vi "数据全参数一起发送整点触发.vi"(6 "数据发送通道":enum16{"TCP", "VISA"}(ring), 8 "PW":string, 9 "MN":string) -> ()   [LabVIEW 2016, in "数据传输系统.lvlib"]
panel:
  out "table":string="提取小时数据"
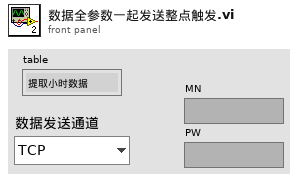
[diagram p1: front panel]
types:
  T1 = typedef "LVDateTimeRec.ctl" = cluster{"秒数的小数部分":dbl, "秒":i32, "分":i32, "时":i32, "日":i32, "月":i32, "年":i32, "天数（周）":i32, "天数（年）":i32, "DST":i32}
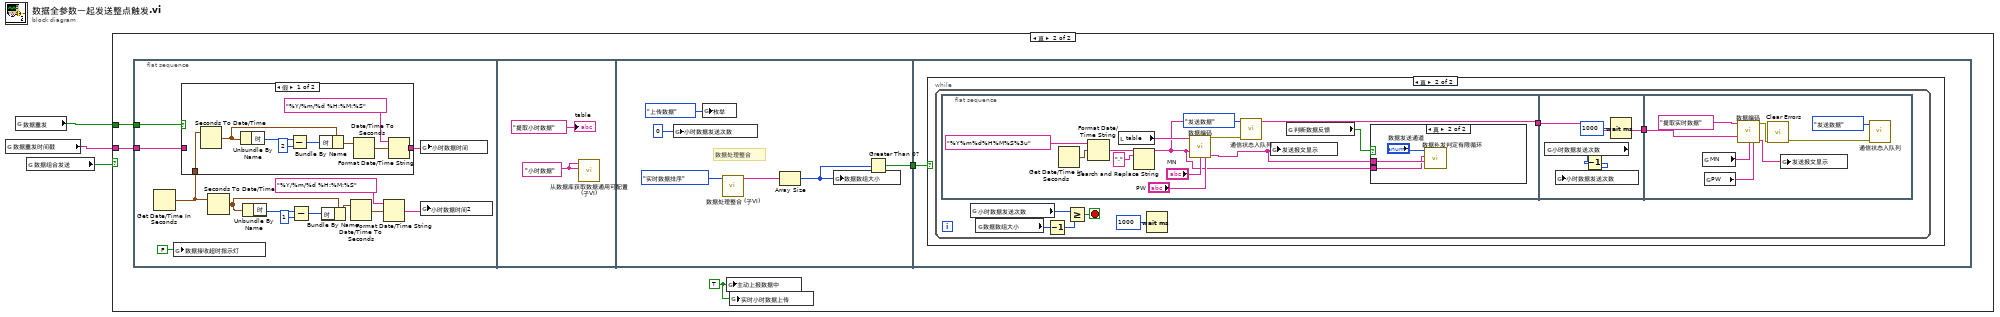
[diagram p0: block diagram]
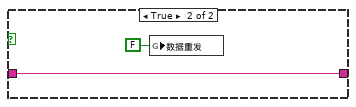
[diagram p3: hidden frame]
diagram:
  n1 = global read "断电保存全局.vi" "数据重发时间戳"() -> (w1:string)
  n2 = global read "断电保存全局.vi" "数据重发"() -> (w2:bool)
  n3 = global read "断电保存全局.vi" "数据组合发送"() -> (w3:bool)
  n4 = case shown="真" w3 {
    tunnel: w2 -> [_ w6]
    tunnel: w1 -> [_ w5]
    frame False {
    }
    frame True {
      w4 = TRUE ("主动上报数据中")
      n5 = flat-sequence {
        tunnel: w6 -> [w15]
        tunnel: w5 -> [w14]
        tunnel: [w35] -> w7
        tunnel: w7 -> [w40]
        frame #0 {
          n6 = Get Date/Time In Seconds() -> (seconds since 1Jan1904=w20:timestamp)
          n7 = global write "全局 数据发送重叠.vi" "数据接收超时指示灯"(FALSE ("数据接收超时指示灯")) -> ()
          n8 = case shown="假" w15 {
            tunnel: w20 -> [w29 _]
            tunnel: [w21 w31] -> w17
            tunnel: w14 -> [_ w31]
            frame False {
              n9 = Seconds To Date/Time(time stamp (now)=w29) -> (date time rec=w24:T1)  [unwired: 1 in]
              n10 = Unbundle By Name(w24) -> ("时"=w22:i32)
              n11 = Subtract(x=w22, y=2) -> (x-y=w25:i32)
              n12 = Bundle By Name(cluster=w24, "时"=w25) -> (w26:T1)
              n13 = Date/Time To Seconds(2:w26) -> (0:w27:timestamp)  [unwired: 1 in]
              n14 = Format Date/Time String(time format string (%c)="%Y/%m/%d %H:%M:%S" ("时间格式字符串(%c)"), seconds (now)=w27) -> (date/time string=w21:string)  [unwired: 1 in]
            }
            frame True {
              n15 = global write "断电保存全局.vi" "数据重发"(FALSE ("数据重发")) -> ()
            }
          }
          n16 = Seconds To Date/Time(time stamp (now)=w20) -> (date time rec=w10:T1)  [unwired: 1 in]
          n17 = Unbundle By Name(w10) -> ("时"=w13:i32)
          n18 = Subtract(x=w13, y=1) -> (x-y=w11:i32)
          n19 = Bundle By Name(cluster=w10, "时"=w11) -> (w9:T1)
          n20 = Date/Time To Seconds(2:w9) -> (0:w19:timestamp)  [unwired: 1 in]
          n21 = Format Date/Time String(time format string (%c)="%Y/%m/%d %H:%M:%S" ("时间格式字符串(%c)"), seconds (now)=w19) -> (date/time string=w16:string)  [unwired: 1 in]
          n22 = global write "全局 时间2.vi" "小时数据时间2"(w16) -> ()
          n23 = global write "全局 水样时间.vi" "小时数据时间"(w17) -> ()
        }
        frame #1 {
          w33 = "小时数据" ("名称（未命名）")
          n24 = call "从数据库获取数据通用可配置(子VI).vi"("table输入"=w33, "列队名（唯一）"=w33) -> ()  [unwired: 8 in, 2 out]
          "table" <- "提取小时数据" ("新元素/子数组")
        }
        frame #2 {
          # "数据处理整合"
          n25 = global write "全局 小时数据发送次数.vi" "小时数据发送次数"(0 ("数值")) -> ()
          n26 = global write "全局1.vi" "枚举"(enum16{"返回请求应答", "上传数据", "返回执行结果"}."上传数据" ("枚举")) -> ()
          n27 = call "数据处理整合 (子VI).vi"("枚举"=enum16{"实时数据排序", "小时数据排序"}."实时数据排序") -> ("已排序的数组"=w39:string[])  [unwired: 10 in]
          n28 = Array Size(array=w39) -> (size(s)=w36:i32)
          n29 = global write "全局 数据数组大小.vi" "数据数组大小"(w36) -> ()
          n30 = Greater Than 0?(x=w36) -> (x > 0?=w35:bool)
        }
        frame #3 {
          n31 = case shown="真" w40 {
            frame False {
            }
            frame True {
              n32 = while {
                stop <- w46 stop-if-true
                n33 = flat-sequence {
                  tunnel: [w48] -> w42
                  tunnel: w42 -> [w66]
                  tunnel: [w66] -> w41
                  tunnel: w41 -> [w67]
                  frame #0 {
                    n34 = Get Date/Time In Seconds() -> (seconds since 1Jan1904=w54:timestamp)
                    n35 = Format Date/Time String(time format string (%c)="%Y%m%d%H%M%S%3u" ("时间格式字符串(%c)"), seconds (now)=w54) -> (date/time string=w55:string)  [unwired: 1 in]
                    n36 = local read "table"() -> (w59:string)
                    n37 = Search and Replace String(input string=w55, search string="." ("搜索字符串")) -> (result string=w48:string)  [unwired: 6 in, 3 out]
                    n38 = call "数据编码.vi"("table输入"=w59, "QN"=w48, "MN"="MN", "PW"="PW") -> ("错误常量"=w49:errorcluster, "通讯包字符串"=w51:string)  [unwired: 10 in]
                    n39 = call "通信状态入队列.vi"("错误输入（无错误）"=w49, "枚举"=enum16{"打开连接", "发送数据", "读取数据", "数据处理", "关闭连接"}."发送数据") -> ()  [unwired: 9 in, 1 out]
                    n40 = global write "全局1.vi" "发送报文显示"(w51) -> ()
                    n41 = global read "断电保存全局.vi" "判断数据反馈"() -> (w52:bool)
                    n42 = case shown="真" w52 {
                      tunnel: w51 -> [_ w62]
                      tunnel: w48 -> [_ w60]
                      frame False {
                      }
                      frame True {
                        n43 = call "数据补发判定有限循环.vi"("数据输入"=w62, "QN"=w60, "数据发送通道"="数据发送通道") -> ()  [unwired: 8 in, 1 out]
                      }
                    }
                  }
                  frame #1 {
                    n44 = global read "全局 小时数据发送次数.vi" "小时数据发送次数"() -> (w64:i32)
                    n45 = Decrement(x=w64) -> (x-1=w63:i32)
                    n46 = global write "全局 小时数据发送次数.vi" "小时数据发送次数"(w63) -> ()
                    n47 = Wait (ms)(milliseconds to wait=u32 1000 ("等待时间（毫秒）")) -> ()  [unwired: 1 out]
                  }
                  frame #2 {
                    n48 = global read "断电保存全局.vi" "MN"() -> (w70:string)
                    n49 = global read "断电保存全局.vi" "PW"() -> (w71:string)
                    n50 = call "数据编码.vi"("table输入"="提取实时数据" ("新元素/子数组"), "QN"=w67, "MN"=w70, "PW"=w71) -> ("错误常量"=w69:errorcluster, "通讯包字符串"=w73:string)  [unwired: 10 in]
                    n51 = call <vilib>:"Clear Errors.vi"("error in (no error)"=w69) -> ("error out"=w68:errorcluster)  [unwired: 5 in, 1 out]
                    n52 = global write "全局1.vi" "发送报文显示"(w73) -> ()
                    n53 = call "通信状态入队列.vi"("错误输入（无错误）"=w68, "枚举"=enum16{"打开连接", "发送数据", "读取数据", "数据处理", "关闭连接"}."发送数据") -> ()  [unwired: 9 in, 1 out]
                  }
                }
                n54 = global read "全局 小时数据发送次数.vi" "小时数据发送次数"() -> (w47:i32)
                n55 = global read "全局 数据数组大小.vi" "数据数组大小"() -> (w43:i32)
                n56 = Decrement(x=w43) -> (x-1=w44:i32)
                n57 = Greater Or Equal?(x=w47, y=w44) -> (x >= y?=w46:bool)
                n58 = Wait (ms)(milliseconds to wait=u32 1000 ("等待时间（毫秒）")) -> ()  [unwired: 1 out]
              }
            }
          }
        }
      }
      n59 = global write "全局 数据发送重叠.vi" "主动上报数据中"(w4) -> ()
      n60 = global write "全局1.vi" "实时小时数据上传"(w4) -> ()
    }
  }
